vi "Write C.vi"(8 "error in (no error)":errorcluster, 10 "C":dbl, 11 "Math Operations in":refnum<class "Math Operations.lvclass">) -> (0 "error out":errorcluster, 3 "Math Operations out":refnum<class "Math Operations.lvclass">)   [LabVIEW 2020, in "Math Operations.lvclass"]
uses:
  Math Operations.lvclass
  Math Operations.lvclass/Math Operations.ctl
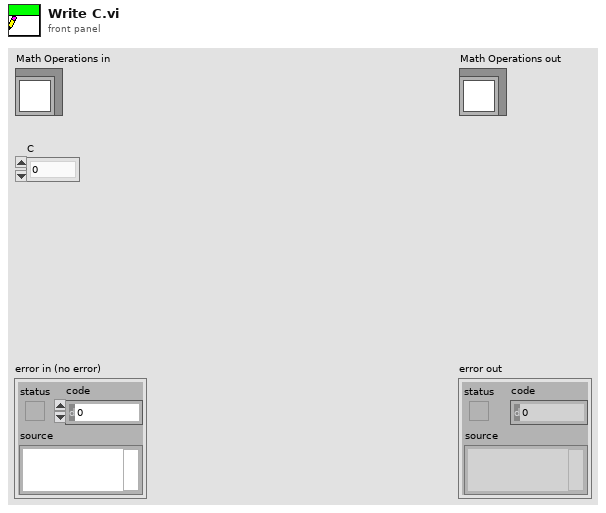
[diagram p1: front panel]
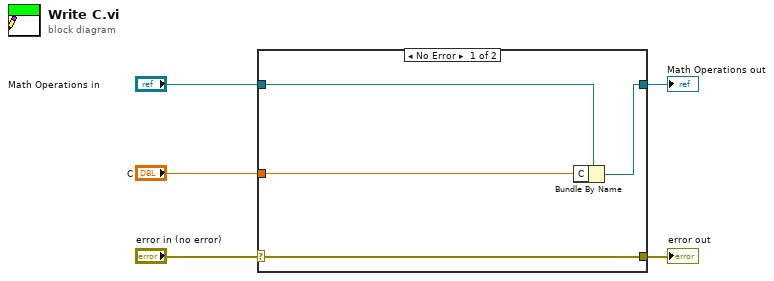
[diagram p0: block diagram]
diagram:
  n1 = case shown="No Error" "error in (no error)" {
    selector: "error in (no error)" -> [w9 w10]
    tunnel: [w9 w10] -> w4
    tunnel: [w7 w11] -> w2
    tunnel: "Math Operations in" -> [w8 w11]
    tunnel: "C" -> [w6 _]
    frame No Error {
      n2 = Bundle By Name(cluster=w8, "C"=w6) -> (w7:refnum<class "Math Operations.lvclass">)
    }
    frame Error {
    }
  }
  "error out" <- w4
  "Math Operations out" <- w2
